vi "ma_align waveforms (common interval with reminder).vi"(0 "Waveform A in":waveform(dbl)={"t0"=timestamp(0 s since 1904-01-01), "dt"=0.0, "Y"=[]}, 5 "Waveform B in":waveform(dbl)={"t0"=timestamp(0 s since 1904-01-01), "dt"=0.0, "Y"=[]}, 11 "error in":errorcluster) -> (4 "Waveform A out":waveform(dbl), 6 "Waveform B out":waveform(dbl), 8 "Reminder Waveform A out":waveform(dbl), 10 "Reminder Waveform B out":waveform(dbl), 15 "error out":errorcluster)   [LabVIEW 2020, in "NI_MAPro.lvlib"]
uses:
  NI_MAPro.lvlib
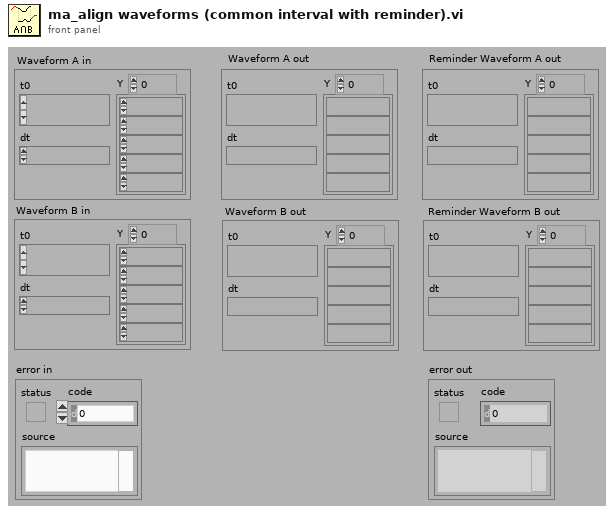
[diagram p1: front panel]
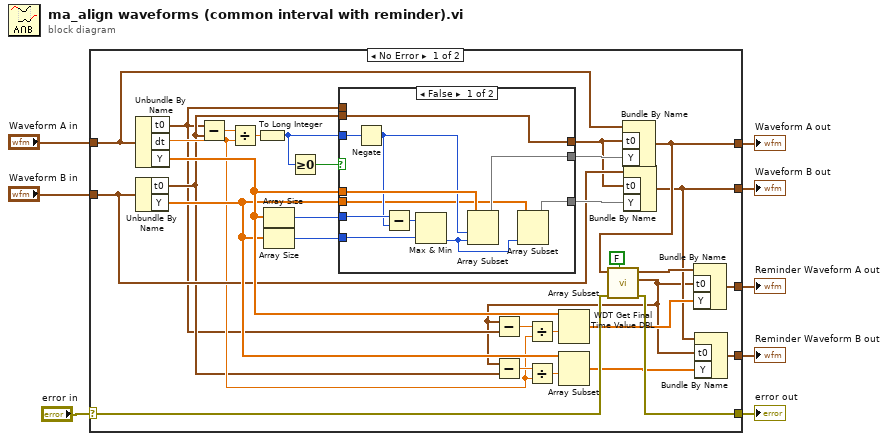
[diagram p0: block diagram]
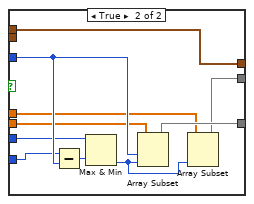
[diagram p2: hidden frame]
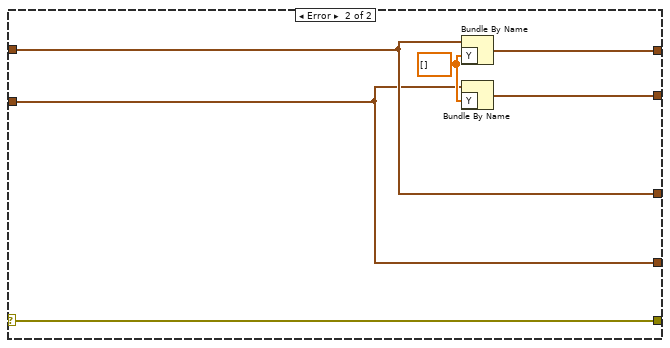
[diagram p3: hidden frame]
diagram:
  n1 = case shown="No Error" "error in" {
    selector: "error in" -> [w25 w66]
    tunnel: [w24 w66] -> w8
    tunnel: [w15 w65] -> w7
    tunnel: [w13 w64] -> w5
    tunnel: "Waveform A in" -> [w18 w62]
    tunnel: "Waveform B in" -> [w17 w61]
    tunnel: [w14 w62] -> w2
    tunnel: [w29 w61] -> w1
    frame No Error {
      n2 = Unbundle By Name(w18) -> ("t0"=w11:timestamp, "dt"=w16:dbl, "Y"=w26:dbl[])
      n3 = Unbundle By Name(w17) -> ("t0"=w12:timestamp, "Y"=w20:dbl[])
      n4 = Subtract(x=w11, y=w12) -> (x-y=w39:dbl)
      n5 = Divide(x=w39, y=w16) -> (x/y=w38:dbl)
      n6 = To Long Integer(number=w38) -> (32bit integer=w37:i32)
      n7 = Array Size(array=w26) -> (size(s)=w33:i32)
      n8 = Array Size(array=w20) -> (size(s)=w32:i32)
      n9 = Greater Or Equal To 0?(x=w37) -> (x >= 0?=w36:bool)
      n10 = case shown="False" w36 {
        tunnel: w37 -> [w50 w59]
        tunnel: w26 -> [w48 w55]
        tunnel: w20 -> [w42 w58]
        tunnel: [w49 w51] -> w9
        tunnel: w11 -> [_ w51]
        tunnel: [w47 w56] -> w35
        tunnel: [w43 w57] -> w34
        tunnel: w12 -> [w49 _]
        tunnel: w33 -> [w46 w52]
        tunnel: w32 -> [w40 w54]
        frame False {
          n11 = Negate(x=w50) -> (-x=w45:i32)
          n12 = Subtract(x=w46, y=w45) -> (x-y=w44:i32)
          n13 = Max & Min(x=w44, y=w40) -> (min(x,y)=w41:i32)  [unwired: 1 out]
          n14 = Array Subset(array=w48, index=w45, length=w41) -> (w47:dbl[])
          n15 = Array Subset(array=w42, length=w41) -> (w43:dbl[])  [unwired: 1 in]
        }
        frame True {
          n16 = Subtract(x=w54, y=w59) -> (x-y=w53:i32)
          n17 = Max & Min(x=w52, y=w53) -> (min(x,y)=w60:i32)  [unwired: 1 out]
          n18 = Array Subset(array=w58, index=w59, length=w60) -> (w57:dbl[])
          n19 = Array Subset(array=w55, length=w60) -> (w56:dbl[])  [unwired: 1 in]
        }
      }
      n20 = Bundle By Name(cluster=w18, "t0"=w9, "Y"=w35) -> (w15:waveform(dbl))
      n21 = call "WDT Get Final Time Value DBL.vi"("open interval? (T)"=FALSE, "error in (no error)"=w25, "waveform in"=w15) -> ("error out"=w24:errorcluster, "tf"=w10:timestamp, "waveform out"=w31:waveform(dbl))  [unwired: 6 in]
      n22 = Subtract(x=w10, y=w11) -> (x-y=w28:dbl)
      n23 = Subtract(x=w10, y=w12) -> (x-y=w22:dbl)
      n24 = Divide(x=w28, y=w16) -> (x/y=w27:dbl)
      n25 = Divide(x=w22, y=w16) -> (x/y=w23:dbl)
      n26 = Array Subset(array=w26, index=w27) -> (w21:dbl[])  [unwired: 1 in]
      n27 = Array Subset(array=w20, index=w23) -> (w19:dbl[])  [unwired: 1 in]
      n28 = Bundle By Name(cluster=w17, "t0"=w9, "Y"=w34) -> (w13:waveform(dbl))
      n29 = Bundle By Name(cluster=w31, "t0"=w10, "Y"=w21) -> (w14:waveform(dbl))
      n30 = Bundle By Name(cluster=w13, "t0"=w10, "Y"=w19) -> (w29:waveform(dbl))
    }
    frame Error {
      w63 = dbl[] [] ("Y")
      n31 = Bundle By Name(cluster=w62, "Y"=w63) -> (w65:waveform(dbl))
      n32 = Bundle By Name(cluster=w61, "Y"=w63) -> (w64:waveform(dbl))
    }
  }
  "Waveform A out" <- w7
  "error out" <- w8
  "Waveform B out" <- w5
  "Reminder Waveform A out" <- w2
  "Reminder Waveform B out" <- w1
